vi "chkEvntSet.vi"(5 "Description":string, 7 "Acquisition Period":dbl, 8 "error in (no error)":errorcluster, 9 "Current Threshold Value":u16, 10 "Short Description":string, 11 "User Name":string) -> (0 "error out":errorcluster)   [LabVIEW 2019]
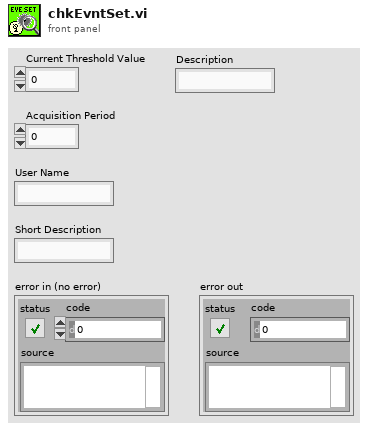
[diagram p1: front panel]
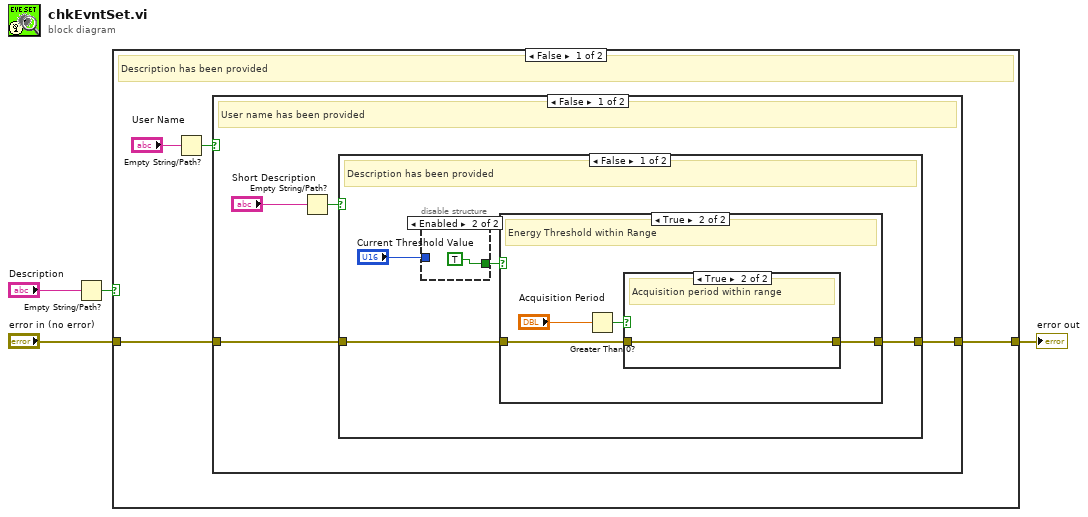
[diagram p0: block diagram]
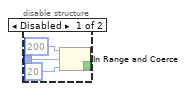
[diagram p2: hidden frame]
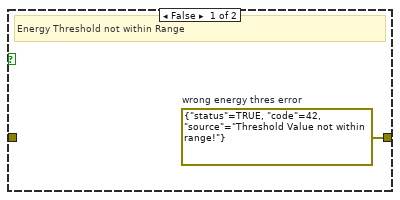
[diagram p3: hidden frame]
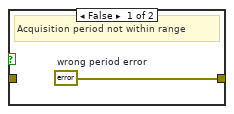
[diagram p4: hidden frame]
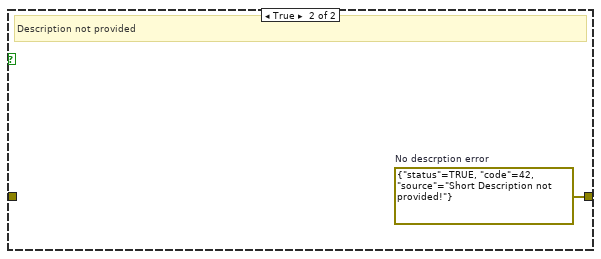
[diagram p5: hidden frame]
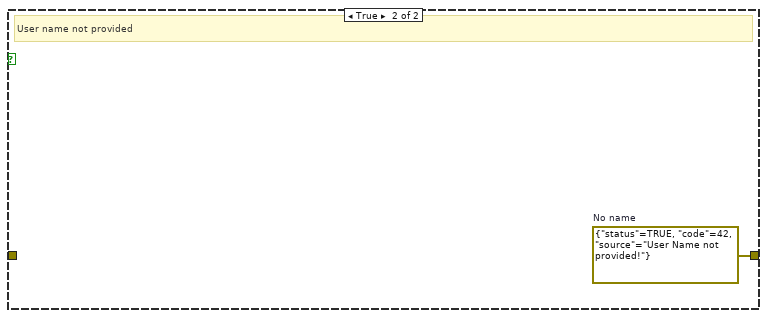
[diagram p6: hidden frame]
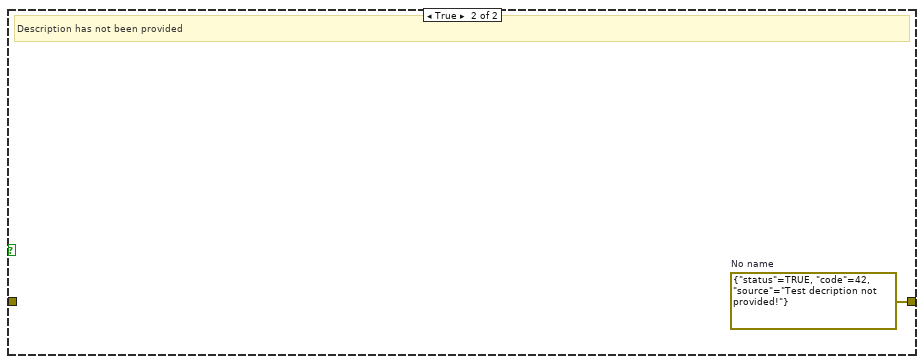
[diagram p7: hidden frame]
diagram:
  n1 = Empty String/Path?(string/path="Description") -> (empty?=w2:bool)
  n2 = case shown="False" w2 {
    tunnel: [w6 w31] -> w4
    tunnel: "error in (no error)" -> [w5 _]
    frame False {
      # "Description has been provided"
      n3 = Empty String/Path?(string/path="User Name") -> (empty?=w8:bool)
      n4 = case shown="False" w8 {
        tunnel: w5 -> [w12 _]
        tunnel: [w11 w30] -> w6
        frame False {
          # "User name has been provided"
          n5 = Empty String/Path?(string/path="Short Description") -> (empty?=w10:bool)
          n6 = case shown="False" w10 {
            tunnel: w12 -> [w16 _]
            tunnel: [w15 w29] -> w11
            frame False {
              # "Description has been provided"
              n7 = disable-structure shown="Enabled" {
                disable-tunnel: [w18 TRUE] -> w14
                disable-tunnel: "Current Threshold Value" -> [w17 _]
                frame Disabled {
                  n8 = In Range and Coerce(upper limit=u16 200 ("lower limit"), x=w17, lower limit=u16 20) -> (In Range?=w18:bool)  [unwired: 1 out]
                }
                frame Enabled {
                }
              }
              n9 = case shown="True" w14 {
                tunnel: w16 -> [_ w25]
                tunnel: [w22 w24] -> w15
                frame False {
                  w22 = errorcluster {"status"=TRUE, "code"=42, "source"="Threshold Value not within range!"}  # wrong energy thres error
                  # "Energy Threshold not within Range"
                }
                frame True {
                  # "Energy Threshold within Range"
                  n10 = Greater Than 0?(x="Acquisition Period") -> (x > 0?=w26:bool)
                  n11 = case shown="True" w26 {
                    tunnel: w25 -> [_ w28]
                    tunnel: [w27 w28] -> w24
                    frame False {
                      w27 = errorcluster {"status"=TRUE, "code"=42, "source"="Acquisition Period not within range!"}  # wrong period error
                      # "Acquisition period not within range"
                    }
                    frame True {
                      # "Acquisition period within range"
                    }
                  }
                }
              }
            }
            frame True {
              w29 = errorcluster {"status"=TRUE, "code"=42, "source"="Short Description not provided!"}  # No descrption error
              # "Description not provided"
            }
          }
        }
        frame True {
          w30 = errorcluster {"status"=TRUE, "code"=42, "source"="User Name not provided!"}  # No name
          # "User name not provided"
        }
      }
    }
    frame True {
      w31 = errorcluster {"status"=TRUE, "code"=42, "source"="Test decription not provided!"}  # No name
      # "Description has not been provided"
    }
  }
  "error out" <- w4
